vi "Teleop Compressor.vi"(11 "Joystick Data":T1) -> ()   [LabVIEW 2013]
uses:
  Joystick Data.ctl
  <vilib>/Rock Robotics/WPI/Relay/WPI_RelayValue.ctl
  Robot Global Data.vi
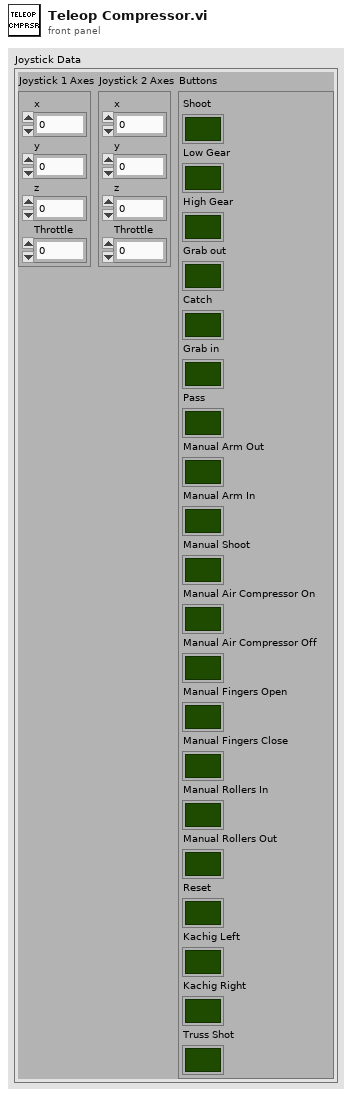
[diagram p1: front panel]
types:
  T1 = typedef "Joystick Data.ctl" = cluster{"Joystick 1 Axes":cluster{"x":dbl, "y":dbl, "z":dbl, "Throttle":dbl}, "Joystick 2 Axes":cluster{"x":dbl, "y":dbl, "z":dbl, "Throttle":dbl}, "Buttons":cluster{"Shoot":bool, "Low Gear":bool, "High Gear":bool, "Grab out":bool, "Catch":bool, "Grab in":bool, "Pass":bool, "Manual Arm Out":bool, "Manual Arm In":bool, "Manual Shoot":bool, "Manual Air Compressor On":bool, "Manual Air Compressor Off":bool, "Manual Fingers Open":bool, "Manual Fingers Close":bool, "Manual Rollers In":bool, "Manual Rollers Out":bool, "Reset":bool, "Kachig Left":bool, "Kachig Right":bool, "Truss Shot":bool}}
  T2 = typedef "WPI_RelayValue.ctl" = enum16{"Off", "On", "Forward", "Reverse"}
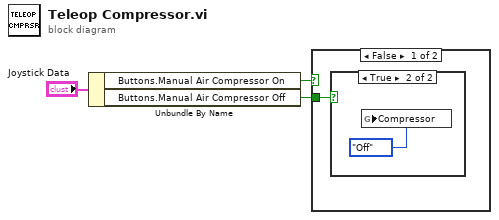
[diagram p0: block diagram]
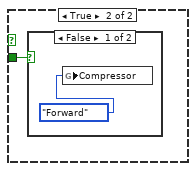
[diagram p3: hidden frame]
diagram:
  n1 = Unbundle By Name("Joystick Data") -> ("Buttons.Manual Air Compressor On"=w2:bool, "Buttons.Manual Air Compressor Off"=w1:bool)
  n2 = case shown="False" w2 {
    tunnel: w1 -> [w4 w6]
    frame False {
      n3 = case shown="True" w4 {
        frame False {
        }
        frame True {
          n4 = global write "Robot Global Data.vi" "Compressor"(WPI_RelayValue."Off" ("Compressor")) -> ()
        }
      }
    }
    frame True {
      n5 = case shown="False" w6 {
        frame False {
          n6 = global write "Robot Global Data.vi" "Compressor"(WPI_RelayValue."Forward" ("Compressor")) -> ()
        }
        frame True {
        }
      }
    }
  }
